vi "FeedbackDecode_CopyLocalFiles.vi"(3 "DataFolder":string, 4 "DataDir":string, 5 "Mode":enum16{"Decode", "Encode"}(ring)) -> (0 "OrigName":string, 2 "MLName":string)   [LabVIEW 2020]
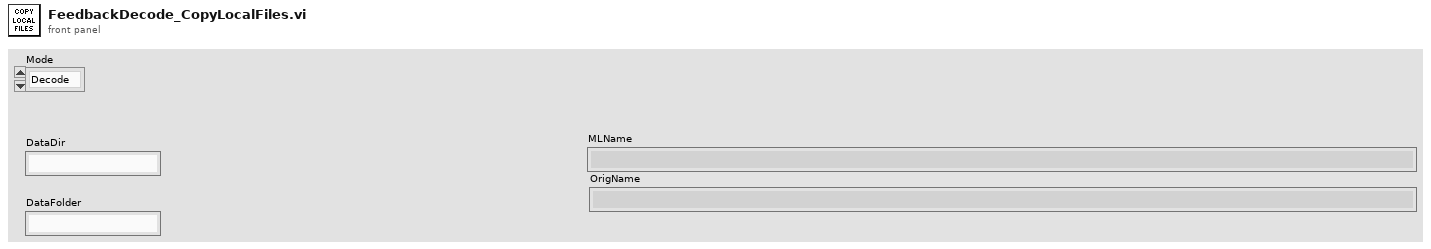
[diagram p1: front panel]
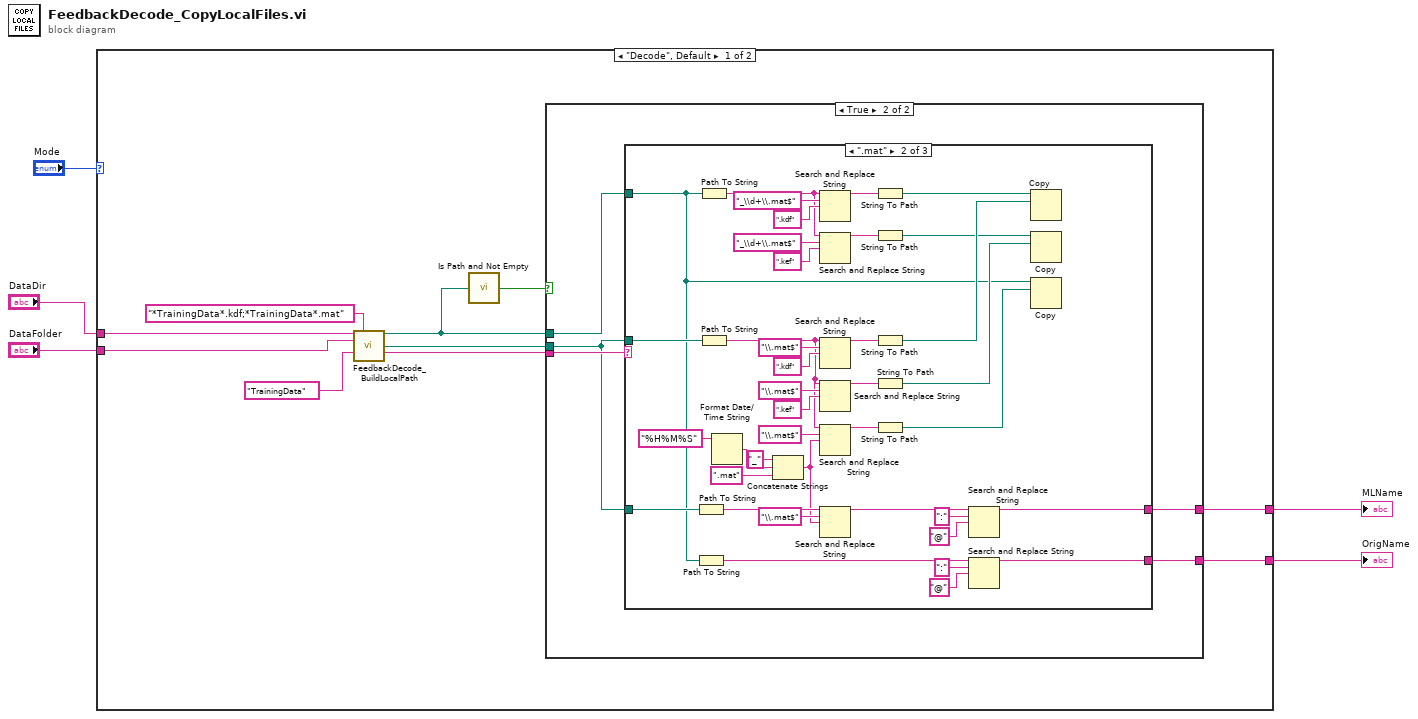
[diagram p0: block diagram]
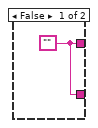
[diagram p2: hidden frame]
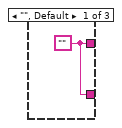
[diagram p3: hidden frame]
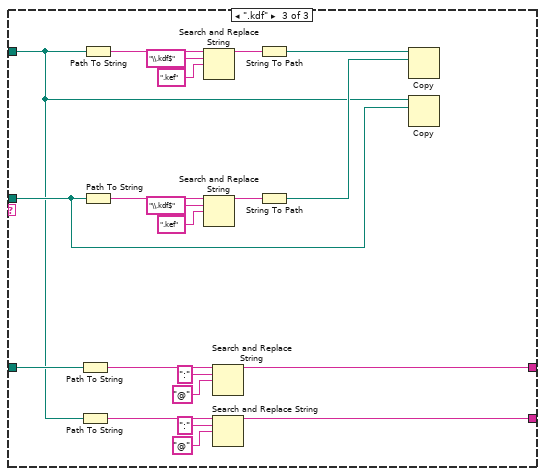
[diagram p4: hidden frame]
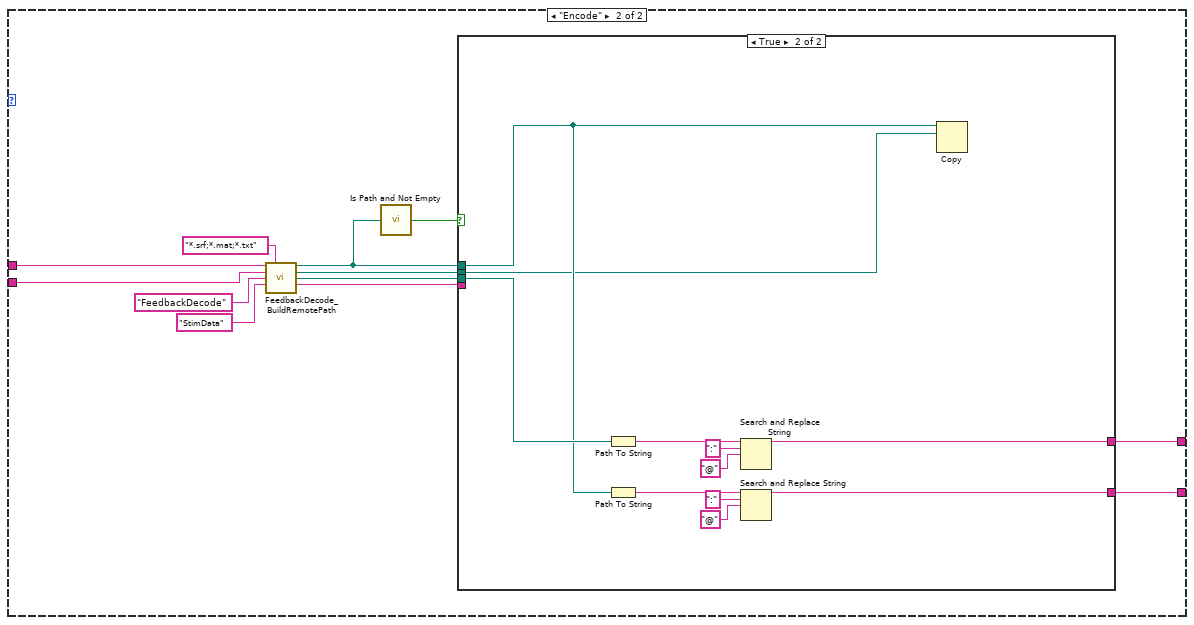
[diagram p5: hidden frame]
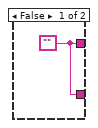
[diagram p6: hidden frame]
diagram:
  n1 = case shown="\"Decode\", Default" "Mode" {
    tunnel: [w10 w87] -> w5
    tunnel: [w9 w86] -> w4
    tunnel: "DataDir" -> [w7 w84]
    tunnel: "DataFolder" -> [w6 w83]
    frame "Decode", Default {
      n2 = call "FeedbackDecode_BuildLocalPath.vi"("DataDir"=w7, "FilePattern"="*TrainingData*.kdf;*TrainingData*.mat" ("pattern (all files)"), "DataFolder"=w6, "HeaderName"="TrainingData" ("TaskName")) -> ("OriginalName"=w11:path, "NewLocalName"=w12:path, "FileExt"=w13:string)  [unwired: 8 in, 1 out]
      n3 = call <vilib>:"Is Path and Not Empty.vi"("path"=w11) -> ("Is Path and Not Empty?"=w8:bool)  [unwired: 4 in]
      n4 = case shown="True" w8 {
        tunnel: w13 -> [_ w21]
        tunnel: w12 -> [_ w17]
        tunnel: w11 -> [_ w20]
        tunnel: [w16 w19] -> w10
        tunnel: [w16 w18] -> w9
        frame False {
          w16 = ""
        }
        frame True {
          n5 = case shown="\".mat\"" w21 {
            tunnel: w20 -> [_ w29 w64]
            tunnel: w17 -> [_ w43 w68]
            tunnel: w17 -> [_ w38 w72]
            tunnel: [w22 w24 w63] -> w19
            tunnel: [w22 w23 w62] -> w18
            frame "", Default {
              w22 = ""
            }
            frame ".mat" {
              n6 = Path To String(path=w38) -> (string=w27:string)
              n7 = Path To String(path=w29) -> (string=w32:string)
              n8 = Path To String(path=w29) -> (string=w57:string)
              n9 = Path To String(path=w43) -> (string=w42:string)
              n10 = Format Date/Time String(time format string (%c)="%H%M%S") -> (date/time string=w45:string)  [unwired: 2 in]
              n11 = Concatenate Strings("_" ("string"), w45, ".mat" ("string")) -> (w26:string)
              n12 = Search and Replace String(input string=w57, search string="_\\d+\\.mat$" ("regular expression"), replace string=".kdf" ("replace string (\"\")")) -> (result string=w56:string)  [unwired: 5 in, 3 out]
              n13 = Search and Replace String(input string=w57, search string="_\\d+\\.mat$" ("regular expression"), replace string=".kef" ("replace string (\"\")")) -> (result string=w55:string)  [unwired: 5 in, 3 out]
              n14 = Search and Replace String(input string=w42, search string="\\.mat$" ("regular expression"), replace string=".kdf" ("replace string (\"\")")) -> (result string=w54:string)  [unwired: 5 in, 3 out]
              n15 = Search and Replace String(input string=w42, search string="\\.mat$" ("regular expression"), replace string=".kef" ("replace string (\"\")")) -> (result string=w49:string)  [unwired: 5 in, 3 out]
              n16 = Search and Replace String(input string=w42, search string="\\.mat$" ("regular expression"), replace string=w26) -> (result string=w46:string)  [unwired: 5 in, 3 out]
              n17 = Search and Replace String(input string=w27, search string="\\.mat$" ("regular expression"), replace string=w26) -> (result string=w25:string)  [unwired: 5 in, 3 out]
              n18 = String To Path(string=w56) -> (path=w37:path)
              n19 = String To Path(string=w55) -> (path=w35:path)
              n20 = String To Path(string=w54) -> (path=w36:path)
              n21 = String To Path(string=w49) -> (path=w34:path)
              n22 = String To Path(string=w46) -> (path=w33:path)
              n23 = Search and Replace String(input string=w25, search string=":", replace string="@" ("replace string (\"\")")) -> (result string=w24:string)  [unwired: 5 in, 3 out]
              n24 = Search and Replace String(input string=w32, search string=":", replace string="@" ("replace string (\"\")")) -> (result string=w23:string)  [unwired: 5 in, 3 out]
              n25 = Copy(10:w36, 11:w37) -> ()  [unwired: 3 in, 3 out]
              n26 = Copy(10:w34, 11:w35) -> ()  [unwired: 3 in, 3 out]
              n27 = Copy(10:w33, 11:w29) -> ()  [unwired: 3 in, 3 out]
            }
            frame ".kdf" {
              n28 = Path To String(path=w72) -> (string=w71:string)
              n29 = Path To String(path=w64) -> (string=w67:string)
              n30 = Path To String(path=w64) -> (string=w80:string)
              n31 = Path To String(path=w68) -> (string=w75:string)
              n32 = Search and Replace String(input string=w80, search string="\\.kdf$" ("regular expression"), replace string=".kef" ("replace string (\"\")")) -> (result string=w79:string)  [unwired: 5 in, 3 out]
              n33 = Search and Replace String(input string=w75, search string="\\.kdf$" ("regular expression"), replace string=".kef" ("replace string (\"\")")) -> (result string=w78:string)  [unwired: 5 in, 3 out]
              n34 = Search and Replace String(input string=w71, search string=":", replace string="@" ("replace string (\"\")")) -> (result string=w63:string)  [unwired: 5 in, 3 out]
              n35 = Search and Replace String(input string=w67, search string=":", replace string="@" ("replace string (\"\")")) -> (result string=w62:string)  [unwired: 5 in, 3 out]
              n36 = String To Path(string=w79) -> (path=w70:path)
              n37 = String To Path(string=w78) -> (path=w69:path)
              n38 = Copy(10:w69, 11:w70) -> ()  [unwired: 3 in, 3 out]
              n39 = Copy(10:w68, 11:w64) -> ()  [unwired: 3 in, 3 out]
            }
          }
        }
      }
    }
    frame "Encode" {
      n40 = call "FeedbackDecode_BuildRemotePath.vi"("CompName"=w84, "FilePattern"="*.srf;*.mat;*.txt" ("pattern (all files)"), "DataFolder"=w83, "TaskName"="FeedbackDecode", "HeaderName"="StimData" ("TaskName")) -> ("OriginalName"=w88:path, "RemoteNetName"=w90:path, "RemoteLocalName"=w89:path, "FileExt"=w91:string)  [unwired: 6 in, 1 out]
      n41 = call <vilib>:"Is Path and Not Empty.vi"("path"=w88) -> ("Is Path and Not Empty?"=w85:bool)  [unwired: 4 in]
      n42 = case shown="True" w85 {
        tunnel: w91 -> [_ _]
        tunnel: w90 -> [_ w96]
        tunnel: w89 -> [_ w106]
        tunnel: w88 -> [_ w97]
        tunnel: [w95 w105] -> w87
        tunnel: [w95 w104] -> w86
        frame False {
          w95 = ""
        }
        frame True {
          n43 = Path To String(path=w106) -> (string=w101:string)
          n44 = Path To String(path=w97) -> (string=w100:string)
          n45 = Search and Replace String(input string=w101, search string=":", replace string="@" ("replace string (\"\")")) -> (result string=w105:string)  [unwired: 5 in, 3 out]
          n46 = Search and Replace String(input string=w100, search string=":", replace string="@" ("replace string (\"\")")) -> (result string=w104:string)  [unwired: 5 in, 3 out]
          n47 = Copy(10:w96, 11:w97) -> ()  [unwired: 3 in, 3 out]
        }
      }
    }
  }
  "MLName" <- w5
  "OrigName" <- w4
